vi "TextTestRunner_Init.vi"(6 "verbosity (1)":u32=1, 7 "publicEvents":T1, 8 "error in (no error)":errorcluster, 9 "descriptions (true)":bool=TRUE, 10 "stream":refnum<queue>, 11 "TextTestRunner in":refnum<class "TextTestRunner.lvclass">) -> (0 "error out":errorcluster, 3 "TextTestRunner out":refnum<class "TextTestRunner.lvclass">)   [LabVIEW 2013, in "TextTestRunner.lvclass"]
uses:
  TextTestRunner.lvclass
  TestRunner/PublicEvents--Cluster.ctl
  TestResult/resultStatusChanged--Cluster.ctl
  TestResult/resultStatus--enum.ctl
  TestResult/testStarted--Cluster.ctl
  TextTestRunner.lvclass/TextTestRunner.ctl
  TestRunner/TestRunner.lvclass
  Libraries/VITesterUtilities.lvlib
  TestResult/TestResult.lvclass
panel:
  # "JKI VI Tester for LabVIEW\nhttp://jkisoft.com/vi-tester\nCopyright (C) 2007-2009, JKI <info@jkisoft.com>\nALL RIGHTS RESERVED"
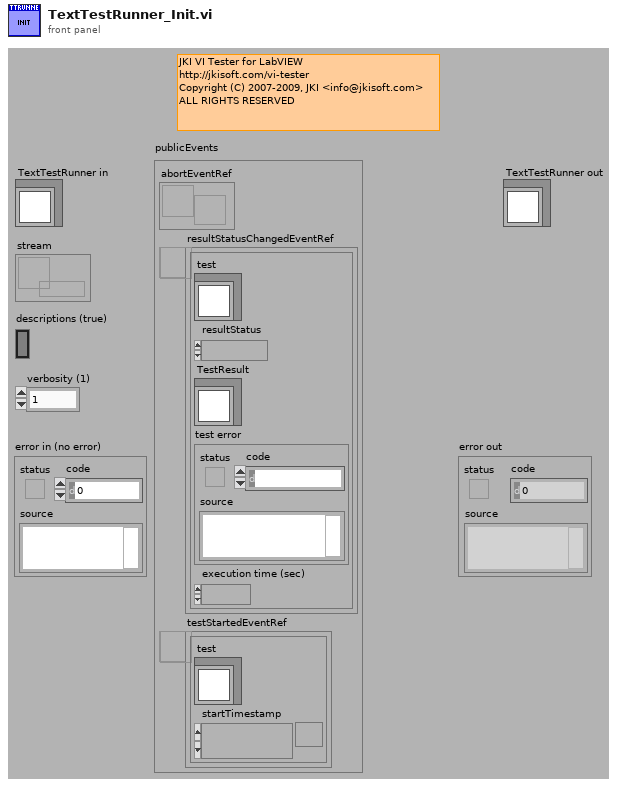
[diagram p1: front panel]
types:
  T1 = typedef "TestRunner.lvclass/PublicEvents--Cluster.ctl" = cluster{"abortEventRef":refnum<user-event>, "resultStatusChangedEventRef":refnum<user-event>, "testStartedEventRef":refnum<user-event>}
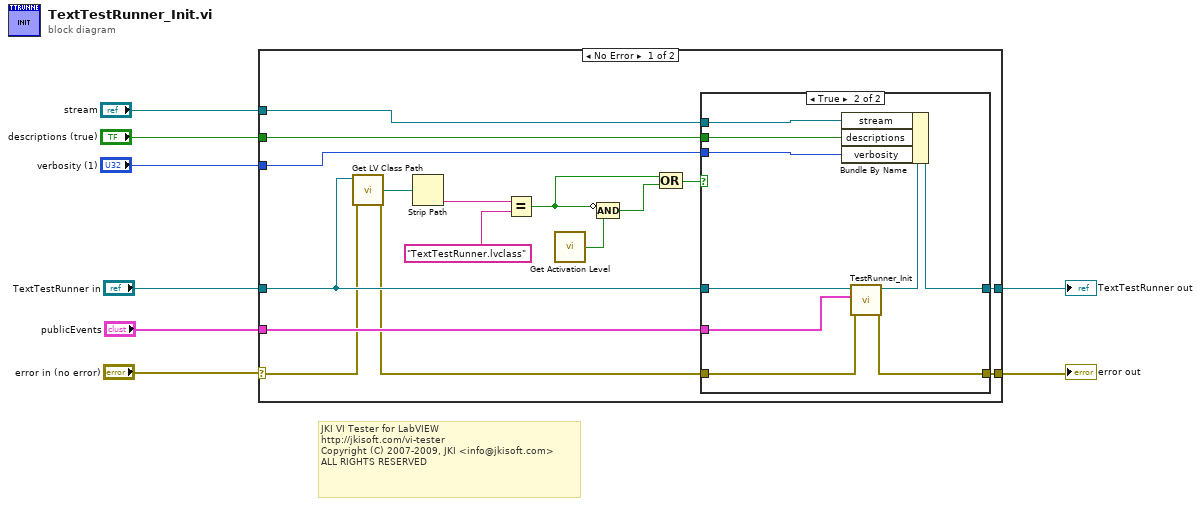
[diagram p0: block diagram]
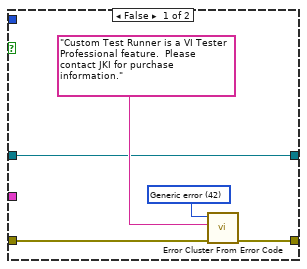
[diagram p2: hidden frame]
diagram:
  # "JKI VI Tester for LabVIEW\nhttp://jkisoft.com/vi-tester\nCopyright (C) 2007-2009, JKI <info@jkisoft.com>\nALL RIGHTS RESERVED"
  n1 = case shown="No Error" "error in (no error)" {
    selector: "error in (no error)" -> [w16 w39]
    tunnel: "TextTestRunner in" -> [w18 w40]
    tunnel: [w24 w40] -> w7
    tunnel: [w20 w39] -> w5
    tunnel: "stream" -> [w23 _]
    tunnel: "descriptions (true)" -> [w22 _]
    tunnel: "verbosity (1)" -> [w21 _]
    tunnel: "publicEvents" -> [w19 _]
    frame No Error {
      n2 = call <vilib>:"Get LV Class Path.vi"("error in (no error)"=w16, "object"=w18) -> ("error out"=w15:errorcluster, "class path"=w17:path)  [unwired: 8 in]
      n3 = Strip Path(path=w17) -> (name=w14:string)  [unwired: 1 out]
      n4 = Equal?(x=w14, y="TextTestRunner.lvclass" ("name")) -> (x = y?=w10:bool)
      n5 = call "Get Activation Level.vi"() -> ("Valid Professional Version"=w12:bool)
      n6 = Compound Arithmetic op=AND(invert w10, w12) -> (w11:bool)
      n7 = Compound Arithmetic op=OR(w10, w11) -> (w9:bool)
      n8 = case shown="True" w9 {
        tunnel: [w25 w38] -> w24
        tunnel: w23 -> [_ w37]
        tunnel: w22 -> [_ w36]
        tunnel: w21 -> [_ w35]
        tunnel: [w26 w33] -> w20
        tunnel: w19 -> [_ w32]
        tunnel: w18 -> [w25 w31]
        tunnel: w15 -> [w27 w30]
        frame False {
          w28 = 42 items=["No error", "Argument error", "Memory is full", "Out of zone", "End of file", "File already open", "Generic file I/O error", "File not found", "File permission error", "Disk is full", "Duplicate path", "Too many files open", "System feature not enabled", "Resource file not found", "Cannot add resource", "Resource not found", "Image not found", "Image memory error", "Pen does not exist", "Config type invalid", "Config token not found", "Config parse error", "Config memory error", "Bad external code format", "Bad external code offset", "External code not present", "Null window", "Destroy window error", "Null menu", "Print aborted", "Bad print record", "Print driver error", "Windows error during printing", "Memory error during printing", "Print dialog error", "Generic print error", "Invalid device refnum", "Device not found", "Device parameter error", "Device unit error", "Cannot open device", "Device call aborted", "Generic error", "Cancelled by user", "Object ID too low", "Object ID too high", "Object not in heap", "Unknown heap", "Unknown object (invalid DefProc)", "Unknown object (DefProc not in table)", "Message out of range", "Invalid (null) method", "Unknown message", "Manager call not supported", "Bad address", "Network operation in progress", "Network operation timed out", "Connection is busy", "Network attribute not supported", "Network error", "Address in use", "System out of memory", "Connection aborted", "Connection refused", "Not connected", "Already connected", "Connection closed", "Initialization error (interapplication manager)", "Bad occurrence", "Wait on unbound occurrence handler", "Occurrence queue overflow", "Datalog type conflict", "Unused", "Unrecognized type (interapplication manager)", "Memory corrupt", "Failed to make temporary DLL", "Old CIN version", "Drag socket not found", "Failed to load drop-object", "Failed to register OLE object", "Failed to release OLE object", "Format specifier type mismatch", "Unknown format specifier", "Too few format specifiers", "Too many format specifiers", "Scan failed", "Newer CIN version", "Error converting to variant", "Runtime menu error", "Password tampered", "Variant attribute not found", "Incompatible variant data type", "Event data is not available", "Event Store is not present", "Occurrence is not found", "Event Queue is not created", "Event info is not available", "Refnum passed is NULL", "Error retrieving Class GUID", "Error retrieving CoClass GUID", "Error retrieving TypeLib GUID.", "Bad built application magic bytes.", "Specific driver is different from the specific driver associated with the Logical Name.", "There is no session opened to the class driver.", "Max Error", "MAX - Error with config objects", "MAX - Error loading configuration", "MAX - Group not supported"]
          n9 = call <vilib>:"Error Cluster From Error Code.vi"("error in (no error)"=w27, "error message (\"\")"="Custom Test Runner is a VI Tester Professional feature.  Please contact JKI for purchase information.", "error code (0)"=w28) -> ("error out"=w26:errorcluster)  [unwired: 6 in]
        }
        frame True {
          n10 = call "TestRunner_Init.vi"("error in (no error)"=w30, "publicEvents"=w32, "TextTestRunner in"=w31) -> ("error out"=w33:errorcluster, "TextTestRunner out"=w34:refnum<class "TextTestRunner.lvclass">)  [unwired: 7 in]
          n11 = Bundle By Name(cluster=w34, "stream"=w37, "descriptions"=w36, "verbosity"=w35) -> (w38:refnum<class "TextTestRunner.lvclass">)
        }
      }
    }
    frame Error {
    }
  }
  "TextTestRunner out" <- w7
  "error out" <- w5
